vi "Motor_askposition.vi"(3 "error in (no error)":errorcluster, 4 "Conversion\n (steps/mm)":dbl[](array[numeric])=[12500.0, 31496.063, 31496.063, 31496.063] format="%#_13g", 5 "reference":refnum<k7>) -> (0 "error out":errorcluster, 1 "position out":dbl[](array[numeric]), 2 "reference out":refnum<k7>)   [LabVIEW 2015]
uses:
  <vilib>/regexp/Match Regular Expression.xnode
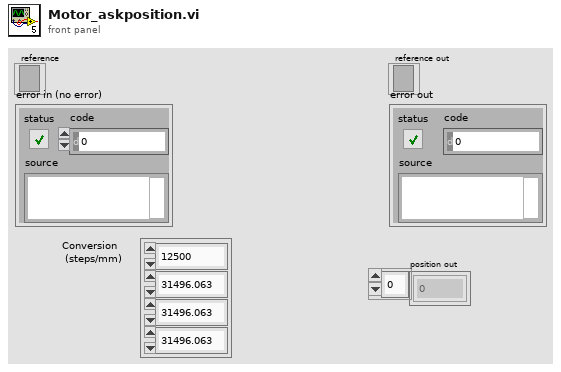
[diagram p1: front panel]
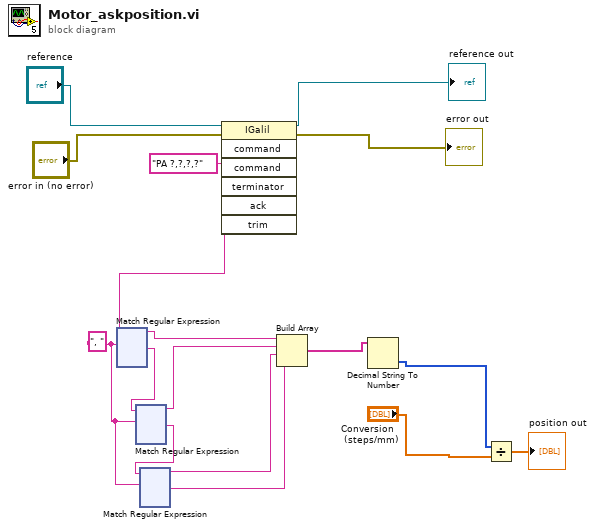
[diagram p0: block diagram]
diagram:
  w3 = ", " ("regular expression")
  n1 = invoke class="IGalil" method="command"(reference="reference", error in="error in (no error)", "command"="PA ?,?,?,?") -> (reference out=→"reference out":refnum<k7>, error out=→"error out":errorcluster, "command"=w5:string)  [unwired: 4 in, 4 out]
  n2 = xnode "Match Regular Expression"("input string"=w5, "regular expression"=w3) -> ("before match"=w16:string, "after match"=w17:string)  [unwired: 4 in, 3 out]
  n3 = xnode "Match Regular Expression"("input string"=w17, "regular expression"=w3) -> ("before match"=w15:string, "after match"=w4:string)  [unwired: 4 in, 3 out]
  n4 = xnode "Match Regular Expression"("input string"=w4, "regular expression"=w3) -> ("before match"=w2:string, "after match"=w1:string)  [unwired: 4 in, 3 out]
  n5 = Build Array(w16, w15, w2, w1) -> (w14:string[])
  n6 = Decimal String To Number(string=w14) -> (number=w11:i32[])  [unwired: 2 in, 1 out]
  n7 = Divide(x=w11, y="Conversion\n (steps/mm)") -> (x/y=→"position out":dbl[])
